vi "M04 Solar Farm.vi"(11 "EV3 in":T1) -> ()   [LabVIEW 2016]
uses:
  <vilib>/NXT/Subs/LVHSConnector.ctl
  <vilib>/NXT/LegoClasses/BrickReference/BrickReference.lvclass
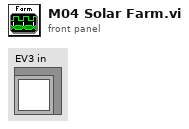
[diagram p1: front panel]
types:
  T1 = typedef "LVHSConnector.ctl" = refnum<class "BrickReference.lvclass">
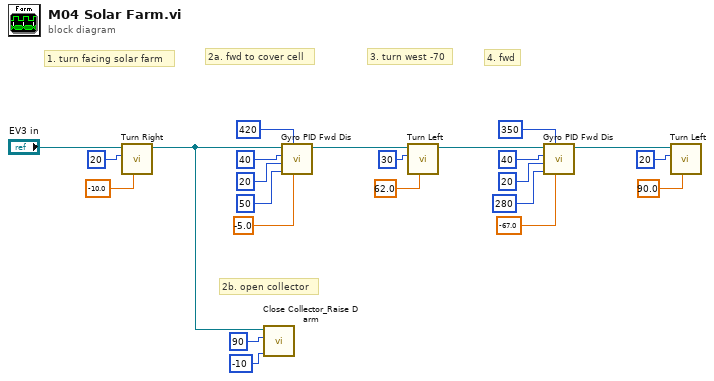
[diagram p0: block diagram]
diagram:
  # "4. fwd"
  # "3. turn west -70"
  # "2b. open collector"
  # "2a. fwd to cover cell"
  # "1. turn facing solar farm"
  n1 = call "Turn Right.vi"("Turning angle"=sgl -10.0, "Motor B (right)"=i8 20, "EV3 in"="EV3 in") -> ("EV3 out"=w1:T1)  [unwired: 8 in]
  n2 = call "Close Collector_Raise D arm.vi"("Power"=i8 -10, "Rotation"=90, "EV3 in"=w1) -> ()  [unwired: 8 in, 1 out]
  n3 = call "Gyro PID Fwd Dis.vi"("Target angle"=sgl -5.0, "Threshold to stop"=420, "Threshold to slow"=50, "Min. speed"=20, "Max. speed"=40, "EV3 in"=w1) -> ("EV3 out"=w13:T1)  [unwired: 5 in]
  n4 = call "Turn Left.vi"("Turning angle"=sgl 62.0, "Motor B (right)"=i8 30, "EV3 in"=w13) -> ("EV3 out"=w8:T1)  [unwired: 8 in]
  n5 = call "Gyro PID Fwd Dis.vi"("Target angle"=sgl -67.0, "Threshold to stop"=350, "Threshold to slow"=280, "Min. speed"=20, "Max. speed"=40, "EV3 in"=w8) -> ("EV3 out"=w4:T1)  [unwired: 5 in]
  n6 = call "Turn Left.vi"("Turning angle"=sgl 90.0, "Motor B (right)"=i8 20, "EV3 in"=w4) -> ()  [unwired: 8 in, 1 out]
